vi "GetParam.vi"(8 "error in (no error)":errorcluster caption="entrée d'erreur (pas d'erreur)", 11 "Roc_Auc_Score.lvclass":refnum<class "Roc_Auc_Score.lvclass">) -> (0 "error out":errorcluster caption="sortie d'erreur", 2 "roc_auc_score":T1={"average"="macro", "sample_weight"=[], "max_fpr"="None", "multi_class"="raise", "labels"=["None"]}, 3 "Roc_Auc_Score.lvclass":refnum<class "Roc_Auc_Score.lvclass">)   [LabVIEW 2020, in "Roc_Auc_Score.lvclass"]
doc: "Get Parameters"
uses:
  Roc_Auc_Score.lvclass
  Roc_Auc_Score.lvclass/Roc_Auc_Score.ctl
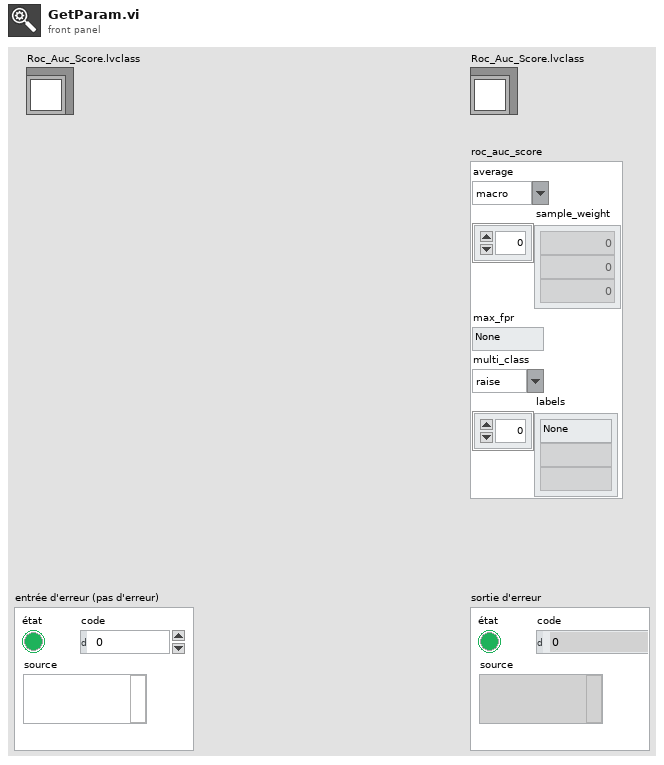
[diagram p1: front panel]
types:
  T1 = cluster{"average":string, "sample_weight":dbl[], "max_fpr":string, "multi_class":string, "labels":string[]}
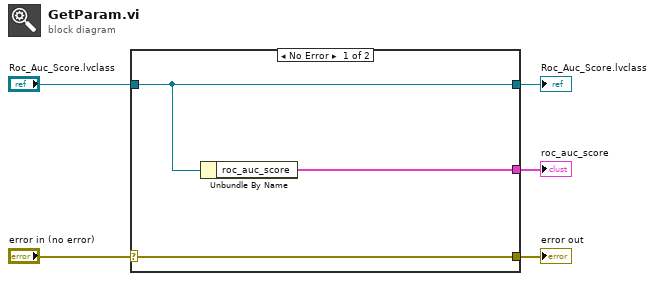
[diagram p0: block diagram]
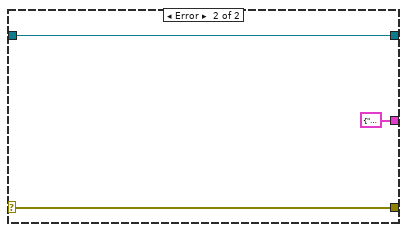
[diagram p2: hidden frame]
diagram:
  n1 = case shown="No Error" "error in (no error)" {
    selector: "error in (no error)" -> [w8 w10]
    tunnel: [w8 w10] -> w4
    tunnel: [w7 w11] -> w2
    tunnel: "Roc_Auc_Score.lvclass" -> [w7 w11]
    tunnel: [w6 T1 {"average"="", "sample_weight"=[], "max_fpr"="", "multi_class"="", "labels"=[]} ("roc_auc_score")] -> w1
    frame No Error {
      n2 = Unbundle By Name(w7) -> ("roc_auc_score"=w6:T1)
    }
    frame Error {
    }
  }
  "error out" <- w4
  "Roc_Auc_Score.lvclass" <- w2
  "roc_auc_score" <- w1
